vi "Find Best XML File In Folder.vi"(7 "folder":path, 8 "error in":errorcluster, 9 "keyword to match (\"\")":string, 10 "desired panel size":T1={"Horizontal"=-1, "Vertical"=-1}, 11 "filename without extension":string) -> (0 "error out":errorcluster, 1 "found?":bool, 2 "panel layout file":path)   [LabVIEW 2012, in "NI_SE_Front Panel Layout.lvlib"]
uses:
  NI_SE_Front Panel Layout.lvlib
  <vilib>/Utility/miscctls.llb/LVPointTypeDef.ctl
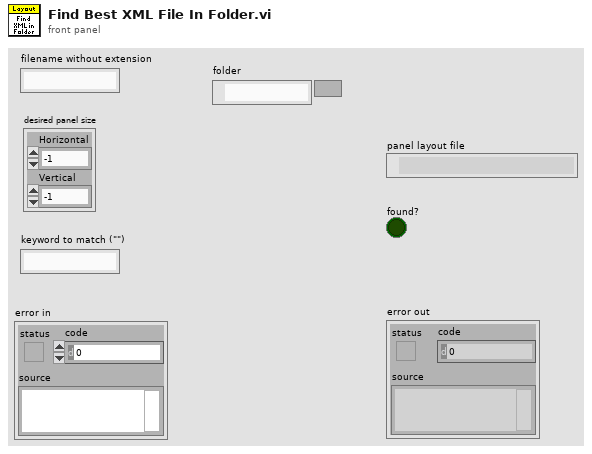
[diagram p1: front panel]
types:
  T1 = typedef "LVPointTypeDef.ctl" = cluster{"Horizontal":i16, "Vertical":i16}
  T2 = typedef "LVRectTypeDef.ctl" = cluster{"Left":i16, "Top":i16, "Right":i16, "Bottom":i16}
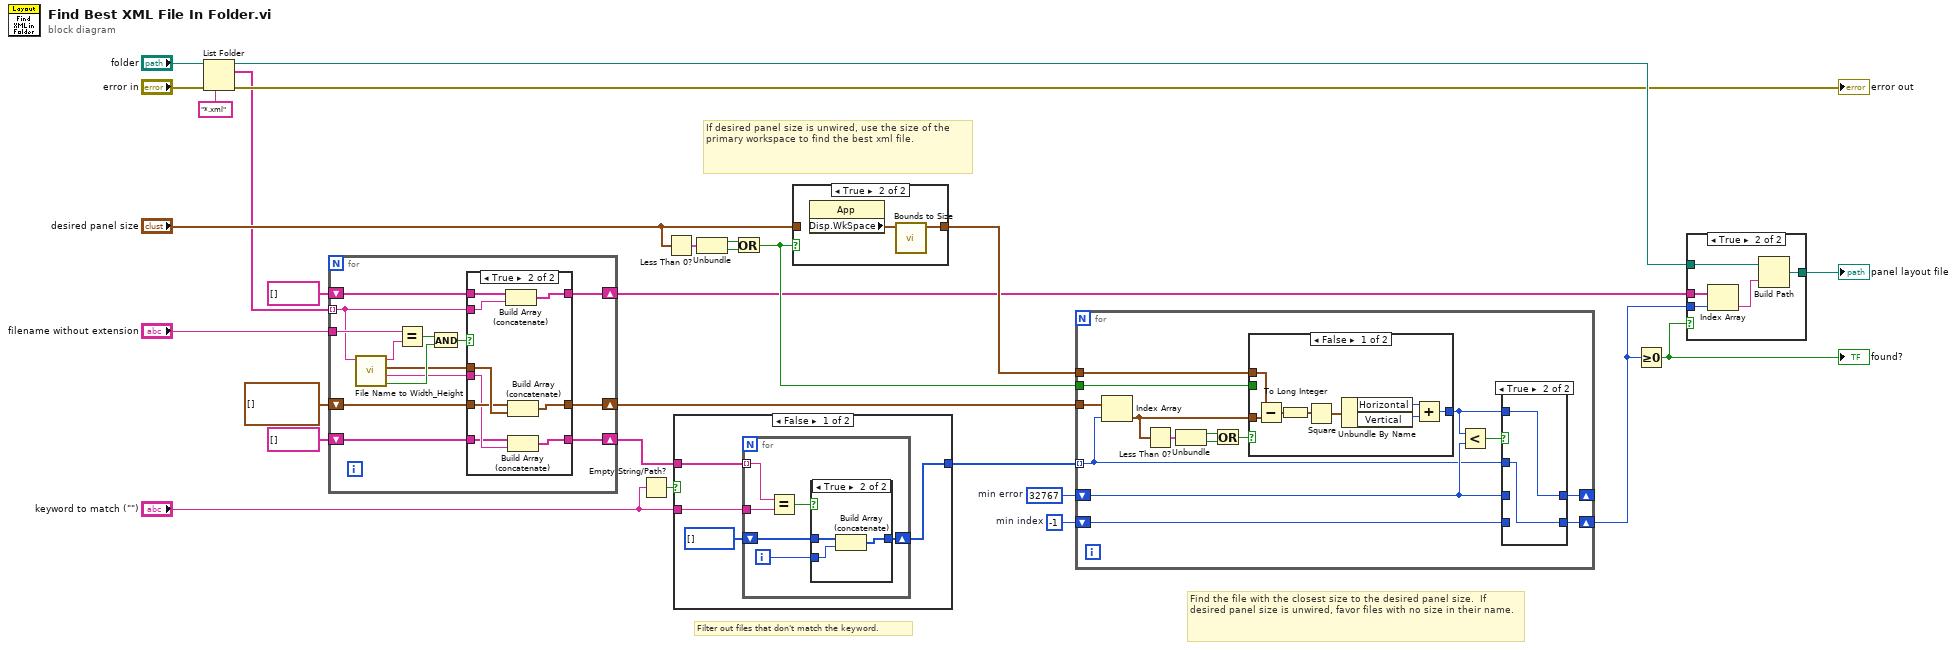
[diagram p0: block diagram]
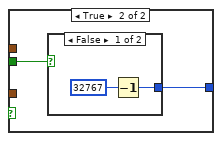
[diagram p2: hidden frame]
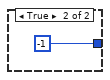
[diagram p3: hidden frame]
diagram:
  w7 = -1  # min index
  w8 = 32767  # min error
  # "Find the file with the closest size to the desired panel size.  If desired panel size is unwired, favor files with no size in their name."
  # "Filter out files that don't match the keyword."
  # "If desired panel size is unwired, use the size of the primary workspace to find the best xml file."
  n1 = List Folder(path="folder", pattern="*.xml", error in="error in") -> (path out=w27:path, filenames=w2:string[], error out=→"error out":errorcluster)  [unwired: 1 in, 1 out]
  n2 = for {
    tunnel: w2 -> [w30] mode=indexing
    tunnel: "filename without extension" -> [w40]
    shift-right: [w34] -> w10
    shift-left: T1[] [] -> [w33]
    shift-right: [w32] -> w14
    shift-left: string[] [] -> [w31]
    shift-right: [w29] -> w1
    shift-left: string[] [] -> [w28]
    n3 = call "File Name to Width_Height.vi"("file name (with xml extension)"=w30) -> ("valid file name?"=w38:bool, "keyword"=w35:string, "size"=w36:T1, "VI file name (no extension)"=w41:string)  [unwired: 7 in]
    n4 = Equal?(x=w40, y=w41) -> (x = y?=w39:bool)
    n5 = And(x=w39, y=w38) -> (x .and. y?=w37:bool)
    n6 = case shown="True" w37 {
      tunnel: w36 -> [_ w53]
      tunnel: w35 -> [_ w50]
      tunnel: [w44 w51] -> w34
      tunnel: w33 -> [w44 w52]
      tunnel: [w43 w49] -> w32
      tunnel: w31 -> [w43 w48]
      tunnel: w30 -> [_ w47]
      tunnel: [w42 w46] -> w29
      tunnel: w28 -> [w42 w45]
      frame False {
      }
      frame True {
        n7 = Build Array (concatenate)(w45, w47) -> (w46:string[])
        n8 = Build Array (concatenate)(w52, w53) -> (w51:T1[])
        n9 = Build Array (concatenate)(w48, w50) -> (w49:string[])
      }
    }
  }
  n10 = Empty String/Path?(string/path="keyword to match (\"\")") -> (empty?=w12:bool)
  n11 = Less Than 0?(x="desired panel size") -> (x < 0?=w18:cluster{"Horizontal":bool, "Vertical":bool})
  n12 = case shown="False" w12 {
    tunnel: w14 -> [w57 w69]
    tunnel: "keyword to match (\"\")" -> [w56 _]
    tunnel: [w54 w68] -> w9
    frame False {
      n13 = for {
        tunnel: w57 -> [w62] mode=indexing
        tunnel: w56 -> [w63]
        shift-right: [w59] -> w54
        shift-left: i32[] [] -> [w58]
        i -> [w60]
        n14 = Equal?(x=w62, y=w63) -> (x = y?=w61:bool)
        n15 = case shown="True" w61 {
          tunnel: w60 -> [_ w67]
          tunnel: [w64 w66] -> w59
          tunnel: w58 -> [w64 w65]
          frame False {
          }
          frame True {
            n16 = Build Array (concatenate)(w65, w67) -> (w66:i32[])
          }
        }
      }
    }
    frame True {
      n17 = for {
        tunnel: w69 -> [_] mode=indexing
        tunnel: [w70] -> w68 mode=indexing
        i -> [w70]
      }
    }
  }
  n18 = Unbundle(w18) -> ("Horizontal"=w19:bool, "Vertical"=w20:bool)
  n19 = Or(x=w19, y=w20) -> (x .or. y?=w4:bool)
  n20 = case shown="True" w4 {
    tunnel: "desired panel size" -> [w71 _]
    tunnel: [w71 w72] -> w5
    frame False {
    }
    frame True {
      n21 = property class="App"() -> ("Disp.WkSpace"=w73:T2)  [unwired: 2 in, 2 out]
      n22 = call "Bounds to Size.vi"("bounds"=w73) -> ("size"=w72:T1)  [unwired: 10 in]
    }
  }
  n23 = for {
    tunnel: w10 -> [w88]
    tunnel: w9 -> [w80] mode=indexing
    tunnel: w5 -> [w83]
    shift-right: [w79] -> _
    shift-left: w8 -> [w82]
    shift-right: [w78] -> w3
    shift-left: w7 -> [w81]
    tunnel: w4 -> [w74]
    n24 = Index Array(array=w88, index=w80) -> (element=w84:T1)
    n25 = Less Than 0?(x=w84) -> (x < 0?=w87:cluster{"Horizontal":bool, "Vertical":bool})
    n26 = Unbundle(w87) -> ("Horizontal"=w86:bool, "Vertical"=w85:bool)
    n27 = Or(x=w86, y=w85) -> (x .or. y?=w75:bool)
    n28 = case shown="False" w75 {
      tunnel: w84 -> [w96 _]
      tunnel: w83 -> [w95 _]
      tunnel: [w90 w98] -> w76
      tunnel: w74 -> [_ w97]
      frame False {
        n29 = Subtract(x=w95, y=w96) -> (x-y=w91:T1)
        n30 = To Long Integer(number=w91) -> (32bit integer=w89:cluster{"Horizontal":i32, "Vertical":i32})
        n31 = Square(x=w89) -> (x^2=w92:cluster{"Horizontal":i32, "Vertical":i32})
        n32 = Unbundle By Name(w92) -> ("Horizontal"=w93:i32, "Vertical"=w94:i32)
        n33 = Add(x=w93, y=w94) -> (x+y=w90:i32)
      }
      frame True {
        n34 = case shown="False" w97 {
          tunnel: [w99 i16 -1] -> w98
          frame False {
            n35 = Decrement(x=i16 32767) -> (x-1=w99:i16)
          }
          frame True {
          }
        }
      }
    }
    n36 = Less?(x=w76, y=w82) -> (x < y?=w77:bool)
    n37 = case shown="True" w77 {
      tunnel: w76 -> [_ w105]
      tunnel: [w103 w105] -> w79
      tunnel: w80 -> [_ w104]
      tunnel: [w102 w104] -> w78
      tunnel: w82 -> [w103 _]
      tunnel: w81 -> [w102 _]
      frame False {
      }
      frame True {
      }
    }
  }
  n38 = Greater Or Equal To 0?(x=w3) -> (x >= 0?=w21:bool)
  "found?" <- w21
  n39 = case shown="True" w21 {
    tunnel: w3 -> [_ w109]
    tunnel: w1 -> [_ w110]
    tunnel: w27 -> [_ w108]
    tunnel: [_ w106] -> w22
    frame False {
    }
    frame True {
      n40 = Index Array(array=w110, index=w109) -> (element=w107:string)
      n41 = Build Path(base path=w108, name or relative path=w107) -> (appended path=w106:path)
    }
  }
  "panel layout file" <- w22
